vi "set_Pos0_exp.vi"(7 "error in (no error)":errorcluster, 9 "Pos0,ps":dbl=-200.0, 10 "Experiment.lvclass in":refnum<class "Experiment.lvclass">) -> (0 "error out":errorcluster, 3 "Experiment.lvclass out":refnum<class "Experiment.lvclass">)   [LabVIEW 2015, in "Experiment.lvclass"]
uses:
  Experiment.lvclass
  Experiment.lvclass/Experiment.ctl
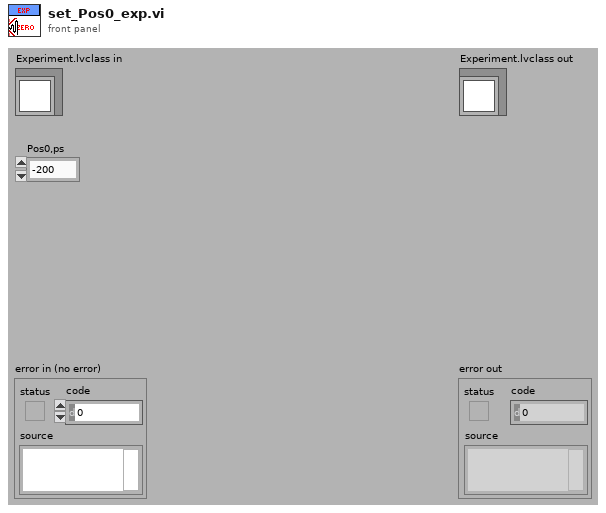
[diagram p1: front panel]
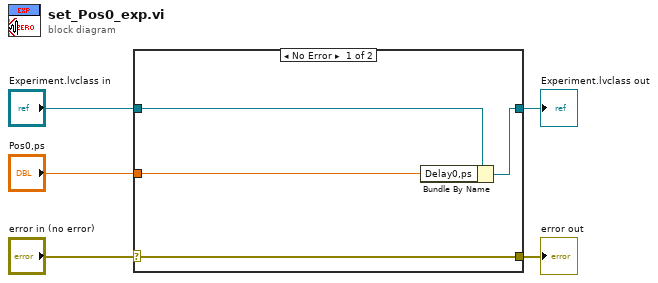
[diagram p0: block diagram]
diagram:
  n1 = case shown="No Error" "error in (no error)" {
    selector: "error in (no error)" -> [w9 w10]
    tunnel: [w9 w10] -> w4
    tunnel: [w7 w11] -> w2
    tunnel: "Experiment.lvclass in" -> [w8 w11]
    tunnel: "Pos0,ps" -> [w6 _]
    frame No Error {
      n2 = Bundle By Name(cluster=w8, "Delay0,ps"=w6) -> (w7:refnum<class "Experiment.lvclass">)
    }
    frame Error {
    }
  }
  "error out" <- w4
  "Experiment.lvclass out" <- w2
